vi "Create Plugins.vi"(8 "error in (no error)":errorcluster, 9 "async plugins tag":string, 10 "inline plugins tag":string, 11 "Application Data In":T1={"Item Tree Control"=refnum, "Top-Level VI"=refnum, "menu reference"=refnum, "queue"=refnum, "Stop Pointer"=refnum, "Buffer Variant"=variant, "Framework Configuration"={"plugins"=[]}, "server ID"=refnum, "framework tag"="", "Values"=refnum, "Hex"=refnum, "ASCII"=refnum, "lines visible"=0, "values padding"=0, "current buffer data"={"decimation"=0, "avg bandwidth"=-1.0, "channels"=[], "byte order"=enum."big-endian", "buffer descriptor"={"buffer type"=enum."Engine", "plugin id"=0, "group id"=0, "transfer id"=0, "offset"=0, "length"=0}, "values channels"={"index"=0, "count"=0, "engine offset"=0}, "select start offset"=18446744073709551615, "select end offset"=0, "channel index"=-1}} {"current buffer data"."channels"."string offset" format="%d bytes"; "current buffer data"."avg bandwidth" format="%.0g bytes"}) -> (0 "error out":errorcluster, 2 "avg bandwidth":dbl, 3 "Application Data out":T1={"Item Tree Control"=refnum, "Top-Level VI"=refnum, "menu reference"=refnum, "queue"=refnum, "Stop Pointer"=refnum, "Buffer Variant"=variant, "Framework Configuration"={"plugins"=[]}, "server ID"=refnum, "framework tag"="", "Values"=refnum, "Hex"=refnum, "ASCII"=refnum, "lines visible"=0, "values padding"=0, "current buffer data"={"decimation"=0, "avg bandwidth"=-1.0, "channels"=[], "byte order"=enum."big-endian", "buffer descriptor"={"buffer type"=enum."Engine", "plugin id"=0, "group id"=0, "transfer id"=0, "offset"=0, "length"=0}, "values channels"={"index"=0, "count"=0, "engine offset"=0}, "select start offset"=18446744073709551615, "select end offset"=0, "channel index"=-1}} {"current buffer data"."channels"."string offset" format="%d bytes"; "current buffer data"."avg bandwidth" format="%.0g bytes"})   [LabVIEW 2017, in "DSF Core.lvlib"]
uses:
  DSF Core.lvlib
  Main VI/Application Data.ctl
  <vilib>/NI/Memory Manager/Classes/Pointer/Pointer.lvclass
  Buffer Reader/Queue Data.ctl
  Buffer Reader/Buffer Data.ctl
  Typedefs/DSF Engine Channel Configuration.ctl
  Typedefs/DSF Data Type.ctl
  Typedefs/DSF Settings Info.ctl
  Typedefs/DSF Byte Order.ctl
  Classes/Thread/Data Server/DSF Buffer Subset Descriptor.ctl
  Typedefs/DSF Buffer Type.ctl
  Main VI/Values Channels.ctl
  Typedefs/DSF Engine Framework Configuration.ctl
  Typedefs/DSF Engine Plugin Configuration.ctl
  Typedefs/DSF Timing Info.ctl
  Typedefs/DSF Engine Plugin Thread Configuration.ctl
  Typedefs/DSF Engine Transfer Group Configuration.ctl
  Typedefs/DSF Direction.ctl
  Typedefs/DSF Engine Transfer Configuration.ctl
  Typedefs/DSF Timeout Behavior.ctl
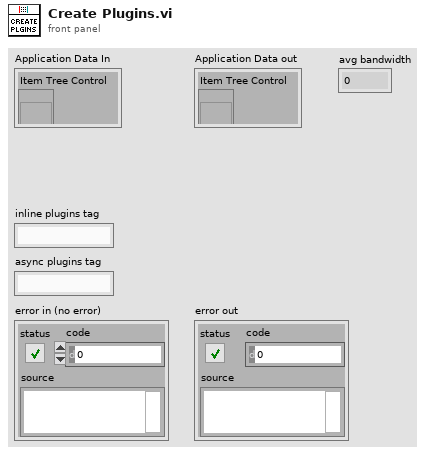
[diagram p1: front panel]
types:
  T1 = typedef "DSF Core.lvlib/Application Data.ctl" = cluster{"Item Tree Control":refnum<vi>, "Top-Level VI":refnum<vi>, "menu reference":refnum<k9>, "queue":refnum<queue>, "Stop Pointer":refnum<class "Pointer.lvclass">, "Buffer Variant":variant, "Framework Configuration":T2, "server ID":refnum<k5>, "framework tag":string, "Values":refnum<vi>, "Hex":refnum<vi>, "ASCII":refnum<vi>, "lines visible":i32, "values padding":i32, "current buffer data":T14}
  T2 = typedef "DSF Core.lvlib/DSF Engine Framework Configuration.ctl" = cluster{"plugins":T3[]}
  T3 = typedef "DSF Core.lvlib/DSF Engine Plugin Configuration.ctl" = cluster{"name":string, "components":string[], "cycle timing":T4, "threads":T5[], "transfer groups":T7[], "settings":T6}
  T4 = typedef "DSF Core.lvlib/DSF Timing Info.ctl" = cluster{"priority":u64, "decimation":u64, "offset":u64}
  T5 = typedef "DSF Core.lvlib/DSF Engine Plugin Thread Configuration.ctl" = cluster{"processor":i32, "priority offset":i16, "settings":T6}
  T6 = typedef "DSF Core.lvlib/DSF Settings Info.ctl" = cluster{"component":string, "name":string, "values":cluster{"key":string, "value":string}[]}[]
  T7 = typedef "DSF Core.lvlib/DSF Engine Transfer Group Configuration.ctl" = cluster{"name":string, "direction":T8, "cycle timing":T4, "thread index":u8, "settings":T6, "transfers":T9[], "timeout behavior":T13, "convert buffers":bool}
  T8 = typedef "DSF Core.lvlib/DSF Direction.ctl" = enum8{"Tx", "Rx"}
  T9 = typedef "DSF Core.lvlib/DSF Engine Transfer Configuration.ctl" = cluster{"name":string, "string byte order":T10, "settings":T6, "channels":T11[]}
  T10 = typedef "DSF Core.lvlib/DSF Byte Order.ctl" = enum8{"big-endian", "little-endian"}
  T11 = typedef "DSF Core.lvlib/DSF Engine Channel Configuration.ctl" = cluster{"string offset":u64, "name":string, "units":string, "engine data type":T12, "string data type":T12, "settings":T6}
  T12 = typedef "DSF Core.lvlib/DSF Data Type.ctl" = enum8{"Bool", "SGL", "DBL", "I8", "I16", "I32", "I64", "U8", "U16", "U32", "U64"}
  T13 = typedef "DSF Core.lvlib/DSF Timeout Behavior.ctl" = enum8{"Increment Late Count", "Throw Error"}
  T14 = typedef "DSF Core.lvlib/Buffer Data.ctl" = cluster{"decimation":u64, "avg bandwidth":dbl, "channels":T11[], "byte order":T10, "buffer descriptor":T15, "values channels":T17, "select start offset":u64, "select end offset":u64, "channel index":i32}
  T15 = typedef "DSF Core.lvlib/DSF Buffer Subset Descriptor.ctl" = cluster{"buffer type":T16, "plugin id":i32, "group id":i32, "transfer id":i32, "offset":u64, "length":i64}
  T16 = typedef "DSF Core.lvlib/DSF Buffer Type.ctl" = enum16{"Engine", "String"}
  T17 = typedef "DSF Core.lvlib/Values Channels.ctl" = cluster{"index":i32, "count":i32, "engine offset":u64}
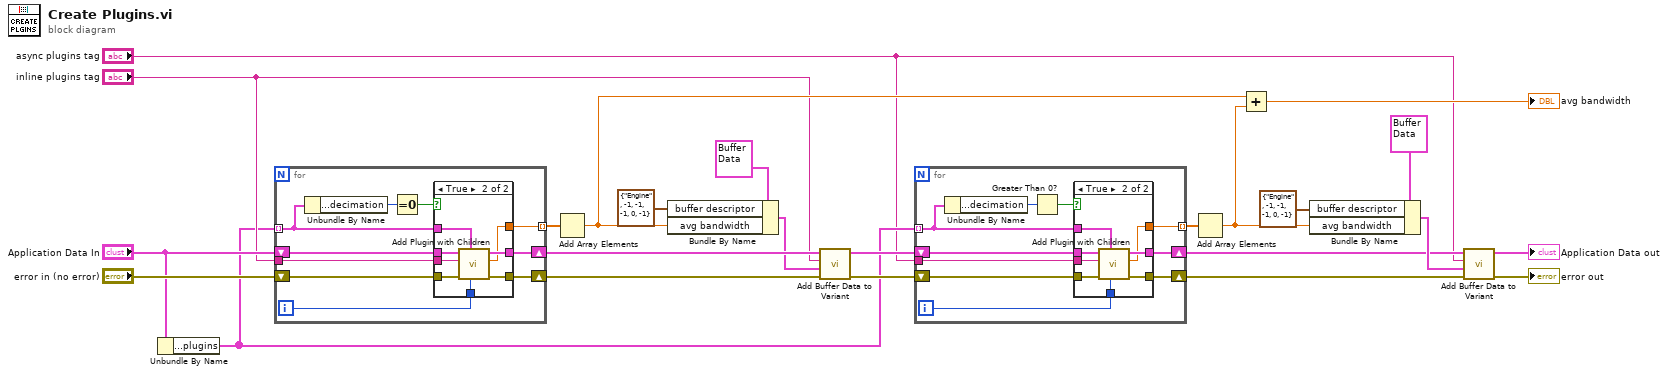
[diagram p0: block diagram]
diagram:
  n1 = Unbundle By Name("Application Data In") -> ("Framework Configuration.plugins"=w2:T3[])
  n2 = for {
    shift-right: [w31] -> w20
    shift-left: "error in (no error)" -> [w33]
    tunnel: "inline plugins tag" -> [w29]
    shift-right: [w32] -> w21
    shift-left: "Application Data In" -> [w34]
    tunnel: [w30] -> w23 mode=indexing
    tunnel: w2 -> [w26] mode=indexing
    i -> [w28]
    n3 = Unbundle By Name(w26) -> ("cycle timing.decimation"=w27:u64)
    n4 = Equal To 0?(x=w27) -> (x = 0?=w25:bool)
    n5 = case shown="True" w25 {
      tunnel: w34 -> [w36 w44]
      tunnel: w33 -> [w35 w43]
      tunnel: [w36 w42] -> w32
      tunnel: [w35 w41] -> w31
      tunnel: [_ w40] -> w30
      tunnel: w29 -> [_ w39]
      tunnel: w28 -> [_ w38]
      tunnel: w26 -> [_ w37]
      frame False {
      }
      frame True {
        n6 = call "Add Plugin with Children.vi"("ID"=w38, "Plugin configuration"=w37, "error in (no error)"=w43, "parent tag"=w39, "Application Data In"=w44) -> ("error out"=w41:errorcluster, "average bandwidth"=w40:dbl, "Application Data Out"=w42:T1)  [unwired: 4 in]
      }
    }
  }
  n7 = Add Array Elements(numeric array=w23) -> (sum=w9:dbl)
  n8 = Bundle By Name(cluster=T14 {"decimation"=0, "avg bandwidth"=0.0, "channels"=[], "byte order"=enum."big-endian", "buffer descriptor"={"buffer type"=enum."Engine", "plugin id"=0, "group id"=0, "transfer id"=0, "offset"=0, "length"=0}, "values channels"={"index"=0, "count"=0, "engine offset"=0}, "select start offset"=18446744073709551615, "select end offset"=0, "channel index"=-1} ("Buffer data"), "buffer descriptor"=T15 {"buffer type"=enum."Engine", "plugin id"=-1, "group id"=-1, "transfer id"=-1, "offset"=0, "length"=-1}, "avg bandwidth"=w9) -> (w17:T14)
  n9 = call "Add Buffer Data to Variant.vi"("error in (no error)"=w20, "Buffer data"=w17, "tag"="inline plugins tag", "Application Data In in"=w21) -> ("error out"=w8:errorcluster, "Application Data In out"=w7:T1)  [unwired: 6 in]
  n10 = for {
    shift-right: [w51] -> w4
    shift-left: w8 -> [w53]
    tunnel: "async plugins tag" -> [w49]
    shift-right: [w52] -> w5
    shift-left: w7 -> [w54]
    tunnel: [w50] -> w6 mode=indexing
    tunnel: w2 -> [w46] mode=indexing
    i -> [w48]
    n11 = Unbundle By Name(w46) -> ("cycle timing.decimation"=w47:u64)
    n12 = Greater Than 0?(x=w47) -> (x > 0?=w45:bool)
    n13 = case shown="True" w45 {
      tunnel: w54 -> [w56 w64]
      tunnel: w53 -> [w55 w63]
      tunnel: [w56 w62] -> w52
      tunnel: [w55 w61] -> w51
      tunnel: [_ w60] -> w50
      tunnel: w49 -> [_ w59]
      tunnel: w48 -> [_ w58]
      tunnel: w46 -> [_ w57]
      frame False {
      }
      frame True {
        n14 = call "Add Plugin with Children.vi"("ID"=w58, "Plugin configuration"=w57, "error in (no error)"=w63, "parent tag"=w59, "Application Data In"=w64) -> ("error out"=w61:errorcluster, "average bandwidth"=w60:dbl, "Application Data Out"=w62:T1)  [unwired: 4 in]
      }
    }
  }
  n15 = Add Array Elements(numeric array=w6) -> (sum=w15:dbl)
  n16 = Add(x=w9, y=w15) -> (x+y=→"avg bandwidth":dbl)
  n17 = Bundle By Name(cluster=T14 {"decimation"=0, "avg bandwidth"=0.0, "channels"=[], "byte order"=enum."big-endian", "buffer descriptor"={"buffer type"=enum."Engine", "plugin id"=0, "group id"=0, "transfer id"=0, "offset"=0, "length"=0}, "values channels"={"index"=0, "count"=0, "engine offset"=0}, "select start offset"=18446744073709551615, "select end offset"=0, "channel index"=-1} ("Buffer data"), "buffer descriptor"=T15 {"buffer type"=enum."Engine", "plugin id"=-1, "group id"=-1, "transfer id"=-1, "offset"=0, "length"=-1}, "avg bandwidth"=w15) -> (w14:T14)
  n18 = call "Add Buffer Data to Variant.vi"("error in (no error)"=w4, "Buffer data"=w14, "tag"="async plugins tag", "Application Data In in"=w5) -> ("error out"=→"error out":errorcluster, "Application Data In out"=→"Application Data out":T1)  [unwired: 6 in]
